vi "FeedbackDecode_20200902.vi"() -> ()   [LabVIEW 2016] (continued)
        n284 = call "FeedbackDecode_PlotHeatmap.vi"("Range"=w3234, "GridIntensity"=w3245, "Instance"=1, "Mode"=w3251) -> ("Pic"=w3236:picture)  [unwired: 2 in, 1 out]
        n285 = call "FeedbackDecode_PlotHeatmap.vi"("Range"=w3234, "GridIntensity"=w3238, "Instance"=2, "Mode"=w3251) -> ("Pic"=w3235:picture)  [unwired: 2 in, 1 out]
        n286 = local write "MedianHM"(w3237) -> ()
        n287 = local write "UlnarHM"(w3236) -> ()
        n288 = local write "EMGHM"(w3235) -> ()
        n289 = for {
          tunnel: w3178 -> [w3331] mode=indexing
          tunnel: [w3330] -> w3180 mode=indexing
          tunnel: w3179 -> [w3327]
          tunnel: w3177 -> [w3329] mode=indexing
          tunnel: [w3326] -> w3176 mode=indexing
          n290 = Build Array(w3331) -> (w3332:dbl[])
          n291 = Build Array(w3329) -> (w3328:dbl[])
          n292 = Bundle By Name("Y"=w3332, "t0"=w3327) -> (w3330:waveform(dbl))  [unwired: 1 in]
          n293 = Bundle By Name("Y"=w3328, "t0"=w3327) -> (w3326:waveform(dbl))  [unwired: 1 in]
        }
        "TASKA Pressure" <- w3180
        "TASKA IR" <- w3176
        n294 = global read "FeedbackDecode_Globals.vi" "FD_PupilClust"() -> (→"PupilClust":T11)
        n295 = case shown="True" w3183 {
          frame False {
          }
          frame True {
            n296 = call <vilib>:"Play Sound File.vi"("path"=path "C:/Windows/Media/Windows Critical Stop.wav") -> ()  [unwired: 9 in, 2 out]
          }
        }
        n297 = local read "CurrMvnt"() -> (w3317:T1)
        n298 = local read "MSMSSphere"() -> (w3270:dbl[][])
        n299 = local read "BaseCnt3"() -> (w3186:i64)
        n300 = local read "LoopCnt"() -> (w3210:u64)
        n301 = case shown="\"Training\"" w3207 {
          tunnel: w3231 -> [_ _ w3412]
          tunnel: [T26 {"[0]"=0.0, "[1]"=0.0, "[2]"=0.0, "[3]"=0.0, "[4]"=0.0, "[5]"=0.0, "[6]"=0.0, "[7]"=0.0, "[8]"=0.0, "[9]"=0.0, "[10]"=0.0, "[11]"=0.0} ("Kinematics") w3411 w3412] -> w3266
          tunnel: w3232 -> [_ w3411 _]
          frame "Off" {
          }
          frame "Training" {
          }
          frame "Decode", Default {
          }
        }
        n302 = local read "MSMSMvnt"() -> (w3271:dbl[])
        n303 = Unbundle By Name(w3317) -> ("Radius"=w3172:dbl)
        n304 = Equal?(x=w3210, y=w3186) -> (x = y?=w3211:bool)
        n305 = Replace Array Subset(array=w3270, new element=w3312, index (row)=0 ("disabled index (row)"), index (col)=0 ("disabled index (col)")) -> (w3174:dbl[][])
        n306 = Cluster To Array(cluster=w3266) -> (array=w3230:dbl[])
        n307 = case shown="True" w3211 {
          frame False {
          }
          frame True {
            n308 = local read "PulseStim"() -> (w3355:bool)
            n309 = case shown="True" w3355 {
              frame False {
                n310 = local read "EncodeClust"() -> (w3358:T9)
                n311 = local write "PulseStim"(TRUE ("PulseStim")) -> ()
                n312 = local read "EncodeClust"() -> (w3362:T9)
                n313 = Unbundle By Name(w3358) -> ("Wait Period"=w3359:dbl)
                n314 = Unbundle By Name(w3362) -> ("Pulse"=w3361:bool)
                n315 = local read "LoopCnt"() -> (w3357:u64)
                n316 = expression code="x*100"(w3359) -> (w3360:dbl)
                n317 = case shown="True" w3361 {
                  tunnel: ["SS.PulseStim=1;" ("EventStr") "SS.PulseStim=0;" ("EventStr")] -> w3364
                  frame False {
                  }
                  frame True {
                  }
                }
                n318 = Add(x=w3357, y=w3360) -> (x+y=w3356:dbl)
                n319 = local write "BaseCnt3"(w3356) -> ()
                n320 = local read "DecodeClust"() -> (w3365:T5)
                n321 = Bundle By Name(cluster=w3365, "EventStr"=w3364) -> (w3367:T5)
                n322 = call "FeedbackDecode_MLComCtrl.vi"("DecodeClustIn"=w3367, "Mode"=T19."SendEvent") -> ()  [unwired: 6 in, 4 out]
              }
              frame True {
                n323 = local read "EncodeClust"() -> (w3372:T9)
                n324 = local write "PulseStim"(FALSE ("PulseStim")) -> ()
                n325 = Unbundle By Name(w3372) -> ("Train Period"=w3373:dbl)
                n326 = local read "LoopCnt"() -> (w3371:u64)
                n327 = expression code="x*100"(w3373) -> (w3374:dbl)
                n328 = Add(x=w3371, y=w3374) -> (x+y=w3370:dbl)
                n329 = local read "DecodeClust"() -> (w3377:T5)
                n330 = local write "BaseCnt3"(w3370) -> ()
                n331 = Bundle By Name(cluster=w3377, "EventStr"="SS.PulseStim=1;") -> (w3379:T5)
                n332 = call "FeedbackDecode_MLComCtrl.vi"("DecodeClustIn"=w3379, "Mode"=T19."SendEvent") -> ()  [unwired: 6 in, 4 out]
              }
            }
          }
        }
        n333 = In Range and Coerce(upper limit=1.0, x=w3230, lower limit=-1.0) -> (coerced(x)=w3273:dbl[])  [unwired: 1 out]
        n334 = Unbundle By Name(w3215) -> ("CtrlButtons.HideSphrs"=w3218:bool)
        n335 = Initialize Array(w3172, 6 ("dimension size")) -> (w3170:dbl[])
        n336 = call "FeedbackDecode_InWindowMDim.vi"("Radius"=w3172, "Targ"=w3222, "Pos"=w3273) -> ("Status"=w3265:enum16{"In", "Out"}, "TargStatus"=w3269:i16[], "TargDist"=w3264:dbl[])  [unwired: 1 in, 1 out]
        n337 = case shown="\"Acquire Start\"" w3325 {
          tunnel: w3265 -> [_ w3511 w3584 _]
          frame "Initialize", Default {
            n338 = local read "DecodeClust"() -> (w3423:T5)
            n339 = Unbundle By Name(w3423) -> ("TestType"=w3421:T23, "CtrlButtons.StartTrials"=w3418:bool, "KinSrc"=w3422:T37)
            n340 = Equal?(x=T30."MSMS", y=w3421) -> (x = y?=w3419:bool)
            n341 = And(x=w3419, y=w3418) -> (x .and. y?=w3417:bool)
            n342 = case shown="True" w3417 {
              tunnel: w3422 -> [_ w3424]
              frame False {
              }
              frame True {
                n343 = stacked-sequence {
                  tunnel: w3424 -> [w3431 _]
                  frame #0 {
                    w3433 = enum16{"Initialize", "Reset", "Run"}."Initialize" ("Mode")
                    # "For step targets, the duration of step is set to ART+ARTR and ARD/ETD are a function of the hold and rise times of the movement."
                    n344 = local read "MvntBuilder"() -> (w3428:T6)
                    n345 = Unbundle By Name(w3428) -> ("MvntList"=w3446:T24)
                    n346 = Unbundle By Name(w3428) -> ("TargParams.Gain"=w3435:dbl, "TargParams.Acc"=w3451:dbl, "Mode"=w3447:enum16{"Selected", "Block", "Random"}, "NTrials"=w3449:dbl)
                    n347 = local read "Timing"() -> (w3455:T3)
                    n348 = Array Size(array=w3446) -> (size(s)=w3448:i32)
                    n349 = case shown="\"Block\", Default" w3447 {
                      selector: w3447 -> [_ w3461]
                      tunnel: [w3460 w3465] -> w3429
                      tunnel: w3448 -> [_ w3464]
                      tunnel: w3449 -> [_ w3463]
                      tunnel: [0.0 ("Perc") w3462] -> w3427
                      frame "Selected" {
                        n350 = property on="MvntList" class="Arr (strict)"() -> ("Index Values"=w3459:u32[])  [unwired: 2 in, 2 out]
                        n351 = Index Array(array=w3459) -> (element=w3460:u32)  [unwired: 1 in]
                      }
                      frame "Block", Default {
                        n352 = call "FeedbackDecode_GenRandBlockIdxs2.vi"("Mode"=w3461, "NumTrials"=w3463, "NumIdxs"=w3464) -> ("RandIdx"=w3465:dbl, "Perc"=w3462:dbl)  [unwired: 2 in]
                      }
                    }
                    "NextIdx" <- w3429
                    n353 = local read "LoopPeriod"() -> (w3434:u64)
                    n354 = Unbundle By Name(w3455) -> ("Dur.ART"=w3437:dbl, "Rnd.ARTR"=w3436:dbl)
                    n355 = Index Array(array=w3446, index=w3429) -> (element=w3425:T1)
                    n356 = Bundle By Name(cluster=w3428, "PercTrials"=w3427) -> (w3426:T6)
                    n357 = Unbundle By Name(w3425) -> ("Tracking"=w3440:enum8{"False", "True", "Mixed"})
                    n358 = Add(x=w3437, y=w3436) -> (x+y=w3438:dbl)
                    n359 = local write "CurrMvnt"(w3425) -> ()
                    n360 = Subtract(x=1.0, y=w3451) -> (x-y=w3453:dbl)
                    n361 = call "FeedbackDecode_GenContTarget.vi"("Gain"=w3435, "StepTime (ms)"=w3438, "MvntClust"=w3425, "LoopPeriod (ms)"=w3434, "Mode"=w3433) -> ()  [unwired: 1 in, 4 out]
                    n362 = call "FeedbackDecode_GenContMvnt.vi"("Mode"=w3433, "LoopPeriod"=w3434, "Gain"=w3435, "MvntClust"=w3425) -> ("MaxTimes (ms)"=w3439:T42)  [unwired: 2 in, 2 out]
                    n363 = local read "MvntEvnt"() -> (w3430:refnum<user-event>)
                    n364 = Unbundle By Name(w3439) -> ("Hold"=w3441:dbl, "Rise"=w3445:dbl, "Trial"=w3452:dbl)
                    n365 = Not Equal To 0?(x=w3440) -> (x != 0?=w3442:bool)
                    "Tracking" <- w3442
                    n366 = local write "MvntBuilder"(w3426) -> ()
                    n367 = Generate User Event(user event=w3430, event data cluster=w3429) -> ()  [unwired: 2 in, 2 out]
                    n368 = expression code="2*x"(w3445) -> (w3444:dbl)
                    n369 = Multiply(x=w3452, y=w3453) -> (x*y=w3454:dbl)
                    n370 = case shown="False" w3442 {
                      tunnel: w3455 -> [w3472 w3485]
                      tunnel: [w3471 w3484] -> w3432
                      tunnel: w3441 -> [w3470 _]
                      tunnel: w3444 -> [w3469 _]
                      tunnel: [w3466 w3482] -> w3443
                      tunnel: w3452 -> [w3467 w3482]
                      tunnel: w3431 -> [w3468 _]
                      tunnel: w3454 -> [_ w3481]
                      frame False {
                        n371 = case shown="\"Training\"" w3468 {
                          tunnel: w3472 -> [w3474 w3480]
                          tunnel: [w3474 w3479] -> w3471
                          tunnel: w3470 -> [_ w3478]
                          tunnel: w3469 -> [_ w3477]
                          tunnel: w3467 -> [w3473 w3476]
                          tunnel: [w3473 w3476] -> w3466
                          frame "Off", Default {
                          }
                          frame "Training" {
                            w3475 = u16 0 ("Rnd.ARDR")
                            n372 = Bundle By Name(cluster=w3480, "Rnd.ARDR"=w3475, "Dur.ARD"=w3478, "Dur.ETD"=w3477, "Rnd.ETDR"=w3475) -> (w3479:T3)
                          }
                        }
                      }
                      frame True {
                        n373 = Bundle By Name(cluster=w3485, "Rnd.ARTR"=u16 0, "Dur.ART"=w3482, "Dur.ETD"=w3481) -> (w3484:T3)
                      }
                    }
                    "TrialTime (ms)" <- w3443
                    n374 = local read "PrevIdx"() -> (w3456:dbl)
                    n375 = Not Equal?(x=w3429, y=w3456) -> (x != y?=w3457:bool)
                    n376 = case shown="True" w3457 {
                      tunnel: w3431 -> [_ w3490]
                      tunnel: w3432 -> [w3486 w3489]
                      frame False {
                        n377 = local write "iTiming"(w3486) -> ()
                      }
                      frame True {
                        n378 = case shown="\"Training\"" w3490 {
                          tunnel: w3489 -> [w3491 w3492]
                          frame "Off", Default {
                            n379 = local write "iTiming"(w3491) -> ()
                          }
                          frame "Training" {
                            n380 = Unbundle By Name(w3492) -> ("Dur.ASD"=w3495:dbl)
                            n381 = Multiply(x=w3495, y=u16 2) -> (x*y=w3496:dbl)
                            n382 = Bundle By Name(cluster=w3492, "Dur.ASD"=w3496) -> (w3493:T3)
                            n383 = local write "iTiming"(w3493) -> ()
                          }
                        }
                        n384 = local read "LoopCnt"() -> (w3487:u64)
                        n385 = local write "ResetCorr"(TRUE ("ResetCorr")) -> ()
                        n386 = local write "BaseCnt1"(w3487) -> ()
                      }
                    }
                  }
                  frame #1 {
                    n387 = local write "Outcome"(enum16{"---", "Success", "Failure"}."---" ("Outcome")) -> ()
                    n388 = local read "NextIdx"() -> (w3497:dbl)
                    n389 = local read "LoopCnt"() -> (w3507:u64)
                    n390 = call "FeedbackDecode_RunOnce.vi"("Instance"=0, "Mode"=enum16{"Reset", "Run"}."Reset") -> ()  [unwired: 1 out]
                    n391 = local write "PrevIdx"(w3497) -> ()
                    n392 = call "FeedbackDecode_LoopComp.vi"("LoopCount"=w3507, "Instance"=0, "Mode"=enum16{"Reset", "Run"}."Reset") -> ()  [unwired: 3 in, 2 out]
                    n393 = call "FeedbackDecode_RunOnce.vi"("Instance"=1, "Mode"=enum16{"Reset", "Run"}."Reset") -> ()  [unwired: 1 out]
                    n394 = local write "State"(T16."Acquire Start" ("Current State")) -> ()
                    "TargCnt" <- u64 0 ("TargAcc")
                    "SubCase" <- 0 ("SubCase")
                  }
                }
              }
            }
          }
          frame "Acquire Start" {
            n395 = local read "iTiming"() -> (w3514:T3)
            n396 = Unbundle By Name(w3514) -> ("Dur.ASD"=w3509:dbl, "Rnd.ASDR"=w3513:dbl)
            n397 = Equal To 0?(x=w3509) -> (x = 0?=w3510:bool)
            n398 = case shown="True" w3510 {
              tunnel: [w3515 enum16{"In", "Out"}."In" ("Status")] -> w3512
              tunnel: w3511 -> [w3515 _]
              frame False {
              }
              frame True {
              }
            }
            n399 = case shown="\"In\", Default" w3512 {
              tunnel: w3509 -> [w3518 _]
              tunnel: w3513 -> [w3517 _]
              frame "In", Default {
                n400 = local read "LoopPeriod"() -> (w3526:u64)
                n401 = local read "LoopCnt"() -> (w3523:u64)
                n402 = local read "Timing"() -> (w3519:T3)
                n403 = call "FeedbackDecode_LoopComp.vi"("RandTime"=w3517, "LoopPeriod"=w3526, "SetTime"=w3518, "LoopCount"=w3523, "Instance"=0, "Mode"=enum16{"Reset", "Run"}."Run") -> ("ActualTime"=w3521:u64, "Outcome"=w3520:enum16{"TimeIn", "TimeOut"})
                n404 = Bundle By Name(cluster=w3519, "Act.ASDA"=w3521) -> (w3522:T3)
                n405 = local write "Timing"(w3522) -> ()
                n406 = case shown="\"TimeOut\"" w3520 {
                  frame "TimeIn", Default {
                    n407 = local read "DecodeClust"() -> (w3528:T5)
                    n408 = Unbundle By Name(w3528) -> ("CtrlButtons.ResetTrial"=w3527:bool)
                    n409 = case shown="True" w3527 {
                      frame False {
                      }
                      frame True {
                        n410 = local read "LoopCnt"() -> (w3531:u64)
                        n411 = local write "State"(T16."Finalize" ("Current State")) -> ()
                        n412 = call "FeedbackDecode_RunOnce.vi"("Instance"=0, "Mode"=enum16{"Reset", "Run"}."Reset") -> ()  [unwired: 1 out]
                        n413 = call "FeedbackDecode_LoopComp.vi"("LoopCount"=w3531, "Instance"=0, "Mode"=enum16{"Reset", "Run"}."Reset") -> ()  [unwired: 3 in, 2 out]
                      }
                    }
                  }
                  frame "TimeOut" {
                    n414 = local read "SubCase"() -> (w3535:i32)
                    n415 = case shown="1, Default" w3535 {
                      frame 0 {
                        # "This subcase delays the execution by 1 loop iteration"
                        n416 = local read "DecodeClust"() -> (w3538:T5)
                        n417 = Unbundle By Name(w3538) -> ("CtrlButtons.CalDEKA"=w3537:bool)
                        n418 = local write "SubCase"(1 ("SubCase")) -> ()
                        n419 = case shown="True" w3537 {
                          frame False {
                          }
                          frame True {
                            n420 = property on="HideSphrs" class="Bool (strict)"("Val(Sgnl)"=TRUE ("Value (Signaling)")) -> ()  [unwired: 2 in, 2 out]
                          }
                        }
                      }
                      frame 1, Default {
                        n421 = local read "LoopCnt"() -> (w3554:u64)
                        n422 = local read "LoopCnt"() -> (w3557:u64)
                        n423 = local read "NIPTime"() -> (w3544:dbl)
                        n424 = local read "LoopCnt"() -> (w3549:u64)
                        n425 = call "FeedbackDecode_GenContTarget.vi"("LoopCount"=w3554, "Mode"=enum16{"Initialize", "Reset", "Run"}."Reset") -> ()  [unwired: 4 in, 4 out]
                        n426 = call "FeedbackDecode_GenContMvnt.vi"("Mode"=enum16{"Initialize", "Reset", "Run"}."Reset", "LoopCount"=w3557) -> ()  [unwired: 4 in, 3 out]
                        n427 = local read "LoopCnt"() -> (w3563:u64)
                        n428 = Format Into String(w3549) -> (resulting string=w3541:string)  [unwired: 3 in, 1 out]
                        n429 = call-poly "FeedbackDecode_VariablesToString.vi"("Format"="%0.0f", "ValueIn"=w3544, "FieldName"="NIPTime" ("Key Word")) -> ("StringOut"=w3547:string)  [unwired: 4 in]
                        n430 = local read "EventParamsFID"() -> (w3543:refnum<file>)
                        n431 = Concatenate Strings("TargOn:SS.EventID=" ("string"), w3541) -> (w3546:string)
                        n432 = call "FeedbackDecode_LoopComp.vi"("LoopCount"=w3563, "Instance"=0, "Mode"=enum16{"Reset", "Run"}."Reset") -> ()  [unwired: 3 in, 2 out]
                        n433 = Concatenate Strings(w3546, ";" ("string"), w3547) -> (w3540:string)
                        n434 = call "FeedbackDecode_WriteTextEOL.vi"("text"=w3540, "refnum in"=w3543) -> ()  [unwired: 8 in, 2 out]
                        n435 = local read "DecodeClust"() -> (w3553:T5)
                        n436 = Bundle By Name(cluster=w3553, "EventStr"=w3540) -> (w3551:T5)
                        n437 = local read "LoopCnt"() -> (w3560:u64)
                        n438 = call "FeedbackDecode_MLComCtrl.vi"("DecodeClustIn"=w3551, "Mode"=T19."SendEvent") -> ()  [unwired: 6 in, 4 out]
                        n439 = local write "State"(T16."Acquire Response" ("Current State")) -> ()
                        n440 = call "FeedbackDecode_LoopComp.vi"("LoopCount"=w3560, "Instance"=1, "Mode"=enum16{"Reset", "Run"}."Reset") -> ()  [unwired: 3 in, 2 out]
                      }
                    }
                  }
                }
              }
              frame "Out" {
                n441 = local read "LoopCnt"() -> (w3569:u64)
                n442 = call "FeedbackDecode_LoopComp.vi"("LoopCount"=w3569, "Instance"=0, "Mode"=enum16{"Reset", "Run"}."Reset") -> ()  [unwired: 3 in, 2 out]
                n443 = local read "DecodeClust"() -> (w3566:T5)
                n444 = Unbundle By Name(w3566) -> ("CtrlButtons.ResetTrial"=w3565:bool)
                n445 = case shown="True" w3565 {
                  frame False {
                  }
                  frame True {
                    n446 = call "FeedbackDecode_RunOnce.vi"("Instance"=0, "Mode"=enum16{"Reset", "Run"}."Reset") -> ()  [unwired: 1 out]
                    n447 = local write "State"(T16."Finalize" ("Current State")) -> ()
                  }
                }
              }
            }
          }
          frame "Acquire Response" {
            n448 = local read "Timing"() -> (w3573:T3)
            n449 = local read "iTiming"() -> (w3579:T3)
            n450 = local read "LoopPeriod"() -> (w3575:u64)
            n451 = local read "LoopCnt"() -> (w3578:u64)
            n452 = Unbundle By Name(w3579) -> ("Dur.ART"=w3581:dbl, "Rnd.ARTR"=w3582:dbl)
            n453 = call "FeedbackDecode_LoopComp.vi"("RandTime"=w3582, "LoopPeriod"=w3575, "SetTime"=w3581, "LoopCount"=w3578, "Instance"=1, "Mode"=enum16{"Reset", "Run"}."Run") -> ("ActualTime"=w3583:u64, "Outcome"=w3574:enum16{"TimeIn", "TimeOut"})
            n454 = Bundle By Name(cluster=w3573, "Act.ARTA"=w3583) -> (w3580:T3)
            n455 = local write "Timing"(w3580) -> ()
            n456 = case shown="\"TimeOut\"" w3574 {
              tunnel: w3584 -> [w3585 _]
              frame "TimeIn", Default {
                n457 = case shown="\"Out\"" w3585 {
                  frame "In", Default {
                    n458 = local read "Tracking"() -> (w3586:bool)
                    n459 = case shown="False" w3586 {
                      tunnel: [w3589 w3601] -> w3587
                      frame False {
                        n460 = local read "Timing"() -> (w3588:T3)
                        n461 = local read "iTiming"() -> (w3594:T3)
                        n462 = local read "LoopPeriod"() -> (w3598:u64)
                        n463 = local read "LoopCnt"() -> (w3595:u64)
                        n464 = Unbundle By Name(w3594) -> ("Dur.ARD"=w3592:dbl, "Rnd.ARDR"=w3591:dbl)
                        n465 = call "FeedbackDecode_LoopComp.vi"("RandTime"=w3591, "LoopPeriod"=w3598, "SetTime"=w3592, "LoopCount"=w3595, "Instance"=0, "Mode"=enum16{"Reset", "Run"}."Run") -> ("ActualTime"=w3590:u64, "Outcome"=w3589:enum16{"TimeIn", "TimeOut"})
                        n466 = Bundle By Name(cluster=w3588, "Act.ARDA"=w3590) -> (w3593:T3)
                        n467 = local write "Timing"(w3593) -> ()
                      }
                      frame True {
                        n468 = local read "TargCnt"() -> (w3602:u64)
                        n469 = local read "MvntBuilder"() -> (w3600:T6)
                        n470 = local read "TrialTime (ms)"() -> (w3606:dbl)
                        n471 = local read "LoopPeriod"() -> (w3604:u64)
                        n472 = Increment(x=w3602) -> (x+1=w3603:u64)
                        n473 = Unbundle By Name(w3600) -> ("TargParams.Acc"=w3599:dbl)
                        n474 = Multiply(x=w3603, y=w3604) -> (x*y=w3607:u64)
                        n475 = Multiply(x=w3606, y=w3599) -> (x*y=w3605:dbl)
                        n476 = local write "TargCnt"(w3603) -> ()
                        n477 = Greater Or Equal?(x=w3607, y=w3605) -> (x >= y?=w3608:bool)
                        n478 = Boolean To (0,1)(Boolean=w3608) -> (0, 1=w3601:i16)
                      }
                    }
                    n479 = case shown="0, Default" w3587 {
                      frame 0, Default {
                        # "TimeIn"
                        n480 = local read "DecodeClust"() -> (w3610:T5)
                        n481 = Unbundle By Name(w3610) -> ("CtrlButtons.ResetTrial"=w3609:bool)
                        n482 = call "FeedbackDecode_RunOnce.vi"("Instance"=0, "Mode"=enum16{"Reset", "Run"}."Run") -> ("State"=w3613:enum16{"RunOnce", "Finished"})
                        n483 = case shown="\"RunOnce\", Default" w3613 {
                          tunnel: w3609 -> [_ w3627]
                          frame "RunOnce", Default {
                            n484 = local read "NIPTime"() -> (w3619:dbl)
                            n485 = local read "LoopCnt"() -> (w3625:u64)
                            n486 = Format Into String(w3625) -> (resulting string=w3616:string)  [unwired: 3 in, 1 out]
                            n487 = call-poly "FeedbackDecode_VariablesToString.vi"("Format"="%0.0f", "ValueIn"=w3619, "FieldName"="NIPTime" ("Key Word")) -> ("StringOut"=w3622:string)  [unwired: 4 in]
                            n488 = local read "EventParamsFID"() -> (w3618:refnum<file>)
                            n489 = Concatenate Strings("InTarg:SS.EventID=" ("string"), w3616) -> (w3621:string)
                            n490 = Concatenate Strings(w3621, ";" ("string"), w3622) -> (w3623:string)
                            n491 = call "FeedbackDecode_WriteTextEOL.vi"("text"=w3623, "refnum in"=w3618) -> ()  [unwired: 8 in, 2 out]
                          }
                          frame "Finished" {
                            n492 = case shown="False" w3627 {
                              frame False {
                              }
                              frame True {
                                n493 = local read "LoopCnt"() -> (w3628:u64)
                                n494 = call "FeedbackDecode_LoopComp.vi"("LoopCount"=w3628, "Instance"=0, "Mode"=enum16{"Reset", "Run"}."Reset") -> ()  [unwired: 3 in, 2 out]
                                n495 = local write "State"(T16."Finalize" ("Current State")) -> ()
                                n496 = call "FeedbackDecode_RunOnce.vi"("Instance"=0, "Mode"=enum16{"Reset", "Run"}."Reset") -> ()  [unwired: 1 out]
                              }
                            }
                          }
                        }
                        n497 = call "FeedbackDecode_RunOnce.vi"("Instance"=1, "Mode"=enum16{"Reset", "Run"}."Reset") -> ()  [unwired: 1 out]
                      }
                      frame 1 {
                        # "TimeOut"
                        n498 = local read "LoopCnt"() -> (w3649:u64)
                        n499 = call "FeedbackDecode_LoopComp.vi"("LoopCount"=w3649, "Instance"=1, "Mode"=enum16{"Reset", "Run"}."Reset") -> ()  [unwired: 3 in, 2 out]
                        n500 = call "FeedbackDecode_RunOnce.vi"("Instance"=0, "Mode"=enum16{"Reset", "Run"}."Reset") -> ()  [unwired: 1 out]
                        n501 = local read "LoopCnt"() -> (w3656:u64)
                        n502 = call "FeedbackDecode_LoopComp.vi"("LoopCount"=w3656, "Instance"=0, "Mode"=enum16{"Reset", "Run"}."Reset") -> ()  [unwired: 3 in, 2 out]
                        n503 = local write "State"(T16."Finalize" ("Current State")) -> ()
                        n504 = local read "NIPTime"() -> (w3641:dbl)
                        n505 = local read "LoopCnt"() -> (w3646:u64)
                        n506 = local write "Outcome"(enum16{"---", "Success", "Failure"}."Success" ("Outcome")) -> ()
                        n507 = Format Into String(w3646) -> (resulting string=w3638:string)  [unwired: 3 in, 1 out]
                        n508 = call-poly "FeedbackDecode_VariablesToString.vi"("Format"="%0.0f", "ValueIn"=w3641, "FieldName"="NIPTime" ("Key Word")) -> ("StringOut"=w3644:string)  [unwired: 4 in]
                        n509 = local read "EventParamsFID"() -> (w3640:refnum<file>)
                        n510 = Concatenate Strings("Success:SS.EventID=" ("string"), w3638) -> (w3643:string)
                        n511 = Concatenate Strings(w3643, ";" ("string"), w3644) -> (w3634:string)
                        n512 = call "FeedbackDecode_WriteTextEOL.vi"("text"=w3634, "refnum in"=w3640) -> ()  [unwired: 8 in, 2 out]
                        n513 = local read "DecodeClust"() -> (w3637:T5)
                        n514 = Bundle By Name(cluster=w3637, "EventStr"=w3634) -> (w3635:T5)
                        n515 = call "FeedbackDecode_MLComCtrl.vi"("DecodeClustIn"=w3635, "Mode"=T19."SendEvent") -> ()  [unwired: 6 in, 4 out]
                      }
                    }
                  }
                  frame "Out" {
                    n516 = local read "DecodeClust"() -> (w3659:T5)
                    n517 = Unbundle By Name(w3659) -> ("CtrlButtons.ResetTrial"=w3658:bool)
                    n518 = case shown="True" w3658 {
                      frame False {
                      }
                      frame True {
                        n519 = local write "State"(T16."Finalize" ("Current State")) -> ()
                      }
                    }
                    n520 = local read "LoopCnt"() -> (w3667:u64)
                    n521 = call "FeedbackDecode_LoopComp.vi"("LoopCount"=w3667, "Instance"=0, "Mode"=enum16{"Reset", "Run"}."Reset") -> ()  [unwired: 3 in, 2 out]
                    n522 = call "FeedbackDecode_RunOnce.vi"("Instance"=1, "Mode"=enum16{"Reset", "Run"}."Run") -> ("State"=w3662:enum16{"RunOnce", "Finished"})
                    n523 = call "FeedbackDecode_RunOnce.vi"("Instance"=0, "Mode"=enum16{"Reset", "Run"}."Reset") -> ()  [unwired: 1 out]
                    n524 = case shown="\"RunOnce\", Default" w3662 {
                      frame "RunOnce", Default {
                        n525 = local read "NIPTime"() -> (w3671:dbl)
                        n526 = local read "LoopCnt"() -> (w3677:u64)
                        n527 = Format Into String(w3677) -> (resulting string=w3668:string)  [unwired: 3 in, 1 out]
                        n528 = call-poly "FeedbackDecode_VariablesToString.vi"("Format"="%0.0f", "ValueIn"=w3671, "FieldName"="NIPTime" ("Key Word")) -> ("StringOut"=w3674:string)  [unwired: 4 in]
                        n529 = local read "EventParamsFID"() -> (w3670:refnum<file>)
                        n530 = Concatenate Strings("OutTarg:SS.EventID=" ("string"), w3668) -> (w3673:string)
                        n531 = Concatenate Strings(w3673, ";" ("string"), w3674) -> (w3675:string)
                        n532 = call "FeedbackDecode_WriteTextEOL.vi"("text"=w3675, "refnum in"=w3670) -> ()  [unwired: 8 in, 2 out]
                      }
                      frame "Finished" {
                      }
                    }
                  }
                }
              }
              frame "TimeOut" {
                n533 = local read "LoopCnt"() -> (w3702:u64)
                n534 = local read "LoopCnt"() -> (w3695:u64)
                n535 = call "FeedbackDecode_RunOnce.vi"("Instance"=0, "Mode"=enum16{"Reset", "Run"}."Reset") -> ()  [unwired: 1 out]
                n536 = call "FeedbackDecode_LoopComp.vi"("LoopCount"=w3702, "Instance"=0, "Mode"=enum16{"Reset", "Run"}."Reset") -> ()  [unwired: 3 in, 2 out]
                n537 = call "FeedbackDecode_LoopComp.vi"("LoopCount"=w3695, "Instance"=1, "Mode"=enum16{"Reset", "Run"}."Reset") -> ()  [unwired: 3 in, 2 out]
                n538 = local write "Outcome"(enum16{"---", "Success", "Failure"}."Failure" ("Outcome")) -> ()
                n539 = local write "State"(T16."Finalize" ("Current State")) -> ()
                n540 = local read "NIPTime"() -> (w3687:dbl)
                n541 = local read "LoopCnt"() -> (w3692:u64)
                n542 = Format Into String(w3692) -> (resulting string=w3684:string)  [unwired: 3 in, 1 out]
                n543 = call-poly "FeedbackDecode_VariablesToString.vi"("Format"="%0.0f", "ValueIn"=w3687, "FieldName"="NIPTime" ("Key Word")) -> ("StringOut"=w3690:string)  [unwired: 4 in]
                n544 = local read "EventParamsFID"() -> (w3686:refnum<file>)
                n545 = Concatenate Strings("Failure:SS.EventID=" ("string"), w3684) -> (w3689:string)
                n546 = Concatenate Strings(w3689, ";" ("string"), w3690) -> (w3680:string)
                n547 = call "FeedbackDecode_WriteTextEOL.vi"("text"=w3680, "refnum in"=w3686) -> ()  [unwired: 8 in, 2 out]
                n548 = local read "DecodeClust"() -> (w3683:T5)
                n549 = Bundle By Name(cluster=w3683, "EventStr"=w3680) -> (w3681:T5)
                n550 = call "FeedbackDecode_MLComCtrl.vi"("DecodeClustIn"=w3681, "Mode"=T19."SendEvent") -> ()  [unwired: 6 in, 4 out]
              }
            }
          }
          frame "Finalize" {
            # "End of trial delay"
            n551 = local read "Timing"() -> (w3704:T3)
            n552 = local read "iTiming"() -> (w3708:T3)
            n553 = local read "LoopPeriod"() -> (w3711:u64)
            n554 = local read "LoopCnt"() -> (w3714:u64)
            n555 = Unbundle By Name(w3708) -> ("Dur.ETD"=w3707:dbl, "Rnd.ETDR"=w3706:dbl)
            n556 = call "FeedbackDecode_LoopComp.vi"("RandTime"=w3706, "LoopPeriod"=w3711, "SetTime"=w3707, "LoopCount"=w3714, "Instance"=0, "Mode"=enum16{"Reset", "Run"}."Run") -> ("ActualTime"=w3705:u64, "Outcome"=w3710:enum16{"TimeIn", "TimeOut"})
            n557 = Bundle By Name(cluster=w3704, "Act.ETDA"=w3705) -> (w3709:T3)
            n558 = local write "Timing"(w3709) -> ()
            n559 = case shown="\"TimeOut\"" w3710 {
              frame "TimeIn", Default {
                n560 = call "FeedbackDecode_RunOnce.vi"("Instance"=0, "Mode"=enum16{"Reset", "Run"}."Run") -> ("State"=w3715:enum16{"RunOnce", "Finished"})
                n561 = case shown="\"RunOnce\", Default" w3715 {
                  frame "RunOnce", Default {
                    n562 = local read "DecodeClust"() -> (w3721:T5)
                    n563 = Unbundle By Name(w3721) -> ("CtrlButtons.CalDEKA"=w3720:bool)
                    n564 = case shown="True" w3720 {
                      frame False {
                      }
                      frame True {
                        n565 = property on="HideSphrs" class="Bool (strict)"("Val(Sgnl)"=FALSE ("Value (Signaling)")) -> ()  [unwired: 2 in, 2 out]
                      }
                    }
                    n566 = call "FeedbackDecode_GenContTarget.vi"("LoopCount"=-inf, "Mode"=enum16{"Initialize", "Reset", "Run"}."Reset") -> ()  [unwired: 4 in, 4 out]
                    n567 = local read "Outcome"() -> (w3722:enum16{"---", "Success", "Failure"})
                    n568 = case shown="\"Failure\"" w3722 {
                      frame "---", Default {
                      }
                      frame "Success" {
                        n569 = local read "PSRef"() -> (w3727:refnum<vi>)
                        n570 = call-by-ref "Start Asynchronous Call"(reference=w3727, "Mode"=enum16{"Cue", "Success", "Failure", "Abort"}."Success", "#S"=1000.0, "Fs"=5000.0) -> ()  [unwired: 10 in, 2 out]
                      }
                      frame "Failure" {
                        n571 = local read "PSRef"() -> (w3731:refnum<vi>)
                        n572 = call-by-ref "Start Asynchronous Call"(reference=w3731, "Mode"=enum16{"Cue", "Success", "Failure", "Abort"}."Failure", "#S"=1000.0 ("Volume"), "Fs"=5000.0) -> ()  [unwired: 10 in, 2 out]
                      }
                    }
                  }
                  frame "Finished" {
                  }
                }
              }
              frame "TimeOut" {
                n573 = local read "DecodeClust"() -> (w3741:T5)
                n574 = local read "MvntBuilder"() -> (w3732:T6)
                n575 = local read "CurrMvnt"() -> (w3739:T1)
                n576 = local read "Outcome"() -> (w3743:enum16{"---", "Success", "Failure"})
                n577 = call "FeedbackDecode_UpdateTrialCnt.vi"("DecodeClustIn"=w3741, "CurrMvnt"=w3739) -> ("DecodeClustOut"=w3740:T5)  [unwired: 1 in]
                n578 = Bundle By Name(cluster=w3740, "Outcome"=w3743) -> (w3742:T5)
                n579 = local read "Timing"() -> (w3756:T3)
                n580 = Unbundle By Name(w3732) -> ("TargParams"=w3757:cluster{"Gain":dbl, "Radius":dbl, "Acc":dbl})
                n581 = local read "EncodeClust"() -> (w3746:T9)
                n582 = local read "TrialArray"() -> (w3755:string[])
                n583 = local read "LoopCnt"() -> (w3737:u64)
                n584 = local read "NIPTime"() -> (w3738:dbl)
                n585 = call "FeedbackDecode_FPPNS2NIP.vi"("NIPTime"=w3738, "EncodeClust"=w3746, "LoopCnt"=w3737, "DecodeClust"=w3742, "TrialTiming"=w3756, "TargParams"=w3757, "MvntClust"=w3739) -> ("TrialParams"=w3748:string)  [unwired: 4 in]
                n586 = Match Pattern(string=w3748, regular expression="SS.MvntMat=\\[[-0-9,;\\.]+\\];") -> (match substring=w3753:string)  [unwired: 1 in, 3 out]
                n587 = local read "EventParamsFID"() -> (w3747:refnum<file>)
                n588 = Insert Into Array(array=w3755, new element=w3748) -> (w3754:string[])  [unwired: 1 in]
                n589 = Concatenate Strings("EndTrial:" ("String"), w3753) -> (w3749:string)
                n590 = Bundle By Name(cluster=w3742, "EventStr"=w3749) -> (w3745:T5)
                n591 = local write "TrialArray"(w3754) -> ()
                n592 = Unbundle By Name(w3732) -> ("PercTrials"=w3733:dbl)
                n593 = call "FeedbackDecode_WriteTextEOL.vi"("text"=w3748, "refnum in"=w3747) -> ()  [unwired: 8 in, 2 out]
                n594 = call "FeedbackDecode_MLComCtrl.vi"("DecodeClustIn"=w3745, "Mode"=T19."SendEvent") -> ("DecodeClustOut"=w3744:T5)  [unwired: 6 in, 3 out]
                n595 = Equal?(x=w3733, y=1.0) -> (x = y?=w3734:bool)
                n596 = Unbundle By Name(w3744) -> ("CtrlButtons.ResetTrial"=w3736:bool)
                n597 = case shown="False" w3736 {
                  tunnel: w3744 -> [w3760 w3795]
                  tunnel: w3734 -> [w3761 _]
                  tunnel: w3732 -> [w3759 _]
                  frame False {
                    n598 = case shown="True" w3761 {
                      tunnel: w3759 -> [_ w3766]
                      tunnel: w3760 -> [w3762 w3765]
                      frame False {
                        n599 = local write "DecodeClust"(w3762) -> ()
                      }
                      frame True {
                        n600 = flat-sequence {
                          tunnel: w3766 -> [w3769]
                          tunnel: w3765 -> [w3772]
                          tunnel: [w3771] -> w3764
                          tunnel: [w3770] -> w3763
                          tunnel: w3764 -> [w3782]
                          tunnel: w3763 -> [w3781]
                          frame #0 {
                            n601 = Unbundle By Name(w3769) -> ("Mode"=w3778:enum16{"Selected", "Block", "Random"}, "NTrials"=w3776:dbl, "MvntList"=w3775:T24)
                            n602 = local write "DecodeClust"(w3772) -> ()
                            n603 = Unbundle By Name(w3772) -> ("CtrlButtons.AcqTraining"=w3771:bool, "CtrlButtons.StartTrials"=w3770:bool)
                            n604 = Array Size(array=w3775) -> (size(s)=w3774:i32)
                            n605 = call "FeedbackDecode_GenRandBlockIdxs2.vi"("Mode"=w3778, "Reset"=TRUE, "NumTrials"=w3776, "NumIdxs"=w3774, "CurrIdx"=0.0) -> ("Perc"=w3768:dbl)  [unwired: 1 out]
                            n606 = Bundle By Name(cluster=w3769, "PercTrials"=w3768) -> (w3767:T6)
                            n607 = local write "MvntBuilder"(w3767) -> ()
                          }
                          frame #1 {
                            n608 = Build Array(w3782, w3781) -> (w3780:bool[])
                            n609 = Boolean Array To Number(Boolean array=w3780) -> (number=w3779:u32)
                            n610 = case shown="3" w3779 {
                              frame 0, Default {
                              }
                              frame 1 {
                                n611 = local read "MvntEvnt"() -> (w3783:refnum<user-event>)
                                n612 = property on="AcqTraining" class="Bool (strict)"("Val(Sgnl)"=FALSE ("Value (Signaling)")) -> ()  [unwired: 2 in, 2 out]
                                n613 = Generate User Event(user event=w3783, event data cluster=0.0 ("event data")) -> ()  [unwired: 2 in, 2 out]
                              }
                              frame 2 {
                                n614 = local read "MvntEvnt"() -> (w3786:refnum<user-event>)
                                n615 = property on="StartTrials" class="Bool (strict)"("Val(Sgnl)"=FALSE ("Value (Signaling)")) -> ()  [unwired: 2 in, 2 out]
                                n616 = Generate User Event(user event=w3786, event data cluster=0.0 ("event data")) -> ()  [unwired: 2 in, 2 out]
                              }
                              frame 3 {
                                w3792 = FALSE ("Value (Signaling)")
                                n617 = local read "MvntEvnt"() -> (w3789:refnum<user-event>)
                                n618 = property on="StartTrials" class="Bool (strict)"("Value"=w3792) -> (error out=w3791:errorcluster)  [unwired: 2 in, 1 out]
                                n619 = property on="AcqTraining" class="Bool (strict)"(error in=w3791, "Val(Sgnl)"=w3792) -> ()  [unwired: 1 in, 2 out]
                                n620 = Generate User Event(user event=w3789, event data cluster=0.0 ("event data")) -> ()  [unwired: 2 in, 2 out]
                              }
                            }
                          }
                        }
                      }
                    }
                  }
                  frame True {
                    n621 = Bundle By Name(cluster=w3795, "CtrlButtons.ResetTrial"=FALSE) -> (w3793:T5)
                    n622 = local write "DecodeClust"(w3793) -> ()
                  }
                }
                n623 = local write "State"(T16."Initialize" ("Current State")) -> ()
              }
            }
          }
        }
        n624 = Replace Array Subset(array=w3271, new element=w3273) -> (w3206:dbl[])  [unwired: 1 in]
        n625 = Replace Array Subset(array=w3174, new element=w3170, index (col)=3 ("disabled index (col)")) -> (w3173:dbl[][])  [unwired: 1 in]
        n626 = Replace Array Subset(array=w3173, new element=w3269, index (col)=4 ("disabled index (col)")) -> (w3220:dbl[][])  [unwired: 1 in]
        n627 = local write "Status"(w3265) -> ()
        n628 = local write "MSMSMvnt"(w3206) -> ()
        n629 = local write "TargDist"(w3264) -> ()
        n630 = case shown="True" w3218 {
          tunnel: w3220 -> [w3381 w3385]
          tunnel: [w3380 w3384] -> w3219
          frame False {
            n631 = Replace Array Subset(array=w3381, new element=dbl[] [1.0, 1.0, 1.0, 1.0, 1.0, 1.0] ("new element/subarray"), index (col)=5 ("disabled index (col)")) -> (w3380:dbl[][])  [unwired: 1 in]
          }
          frame True {
            n632 = Replace Array Subset(array=w3385, new element=dbl[] [0.0, 0.0, 0.0, 0.0, 0.0, 0.0] ("new element/subarray"), index (col)=5 ("disabled index (col)")) -> (w3384:dbl[][])  [unwired: 1 in]
          }
        }
        n633 = Unbundle By Name(w3209) -> ("CtrlButtons.ConnDEKA"=w3208:bool, "KMvntClust.CtrlMode"=w3205:T43, "KMvntClust.CtrlSpd"=w3201:sgl[], "KinSrc"=w3199:T37, "DEKAMode"=w3195:enum16{"Velocity", "Position"}, "CtrlButtons.CalDEKA"=w3202:bool)
        n634 = global write "FeedbackDecode_Globals.vi" "FD_MSMSMvnt"(w3206) -> ()
        n635 = call "FeedbackDecode_CombineMSMSPackets.vi"("SphereArray"=w3219, "MvntArray"=w3206) -> ()  [unwired: 1 in]
        n636 = local write "MSMSSphere"(w3219) -> ()
        n637 = case shown="False" w3202 {
          tunnel: w3202 -> [_ w3350]
          frame False {
          }
          frame True {
            n638 = call "FeedbackDecode_RunOnce.vi"("Instance"=2, "Mode"=enum16{"Reset", "Run"}."Run") -> ("State"=w3351:enum16{"RunOnce", "Finished"})
            n639 = case shown="\"RunOnce\", Default" w3351 {
              tunnel: w3350 -> [w3354 _]
              frame "RunOnce", Default {
                n640 = global write "FeedbackDecode_Globals.vi" "FD_CalDEKA"(w3354) -> ()
              }
              frame "Finished" {
              }
            }
          }
        }
        n641 = global write "FeedbackDecode_Globals.vi" "FD_ConnDEKA"(w3208) -> ()
        n642 = global write "FeedbackDecode_Globals.vi" "FD_CtrlMode"(w3205) -> ()
        n643 = global write "FeedbackDecode_Globals.vi" "FD_CtrlSpeed"(w3201) -> ()
        n644 = global write "FeedbackDecode_Globals.vi" "FD_KinSrc"(w3199) -> ()
        n645 = global write "FeedbackDecode_Globals.vi" "FD_DEKAMode"(w3195) -> ()
        n646 = global read "FeedbackDecode_Globals.vi" "FD_Stop"() -> (w3200:bool)
        n647 = node-c288() -> ()  [unwired: 1 in, 1 out]
        "LoopCnt" <- w3318
      }
      n648 = control-ref of="RespStr"() -> (w326:refnum<vi>)
      n649 = call "FeedbackDecode_PickROI.vi"("RespStrRef"=w326) -> ()  [unwired: 3 in]
      n650 = call "FeedbackDecode_PickROI_Adv.vi"("RespStrRef"=w326) -> ()  [unwired: 3 in]
      n651 = local read "PupilTracker"() -> (w325:bool)
      n652 = while {
        stop <- w336 stop-if-true
        n653 = Wait (ms)(milliseconds to wait=u32 1000) -> ()  [unwired: 1 out]
        n654 = local read "DataPath"() -> (w335:path)
        n655 = global read "FeedbackDecode_Globals.vi" "FD_Stop"() -> (w336:bool)
        n656 = call "FeedbackDecode_RecordAV.vi"("FullDataPath"=w335) -> ()  [unwired: 3 in]
      }
      n657 = case shown="True" w325 {
        frame False {
        }
        frame True {
          n658 = while {
            stop <- w330 stop-if-true
            n659 = local read "DataPath"() -> (w329:path)
            n660 = Wait (ms)(milliseconds to wait=u32 1000) -> ()  [unwired: 1 out]
            n661 = global read "FeedbackDecode_Globals.vi" "FD_Stop"() -> (w330:bool)
            n662 = call "FeedbackDecode_GetPupilInfo.vi"("FullDataPath"=w329) -> ()  [unwired: 3 in]
          }
        }
      }
      n663 = while {
        stop <- w339 stop-if-true
        n664 = local read "EvntReg"() -> (w338:refnum<event-registration>)
        n665 = event shown="[12] \"CognitiveLoad.ConnectECG\": Value Change" {
          selector: w338 -> [_ _ _ _ _ _ _ _ _ _ _ _ _ _ _ _ _ _ _ _ _ _ _ _ _ _ _ _ _ _ _ _ _ _ _ _ _ _ _ _ _ _ _ _ _ _ _ _ _ _ _ _ _ _ _ _ _ _ _ _ _ _ _ _ _ _ _ _ _ _ _ _ _ _ _ _ _ _ _ _ _ _ _ _ _ _ _ _ _ _ _ _ _ _ _ _ _ _ _ _ _ _ _ _ _ _ _ _ _ _ _ _]
          dyn-events: _ -> [_ _ _ _ _ _ _ _ _ _ _ _ _ _ _ _ _ _ _ _ _ _ _ _ _ _ _ _ _ _ _ _ _ _ _ _ _ _ _ _ _ _ _ _ _ _ _ _ _ _ _ _ _ _ _ _ _ _ _ _ _ _ _ _ _ _ _ _ _ _ _ _ _ _ _ _ _ _ _ _ _ _ _ _ _ _ _ _ _ _ _ _ _ _ _ _ _ _ _ _ _ _ _ _ _ _ _ _ _ _ _ _]
          timeout: _ -> [_ _ _ _ _ _ _ _ _ _ _ _ _ _ _ _ _ _ _ _ _ _ _ _ _ _ _ _ _ _ _ _ _ _ _ _ _ _ _ _ _ _ _ _ _ _ _ _ _ _ _ _ _ _ _ _ _ _ _ _ _ _ _ _ _ _ _ _ _ _ _ _ _ _ _ _ _ _ _ _ _ _ _ _ _ _ _ _ _ _ _ _ _ _ _ _ _ _ _ _ _ _ _ _ _ _ _ _ _ _ _ _]
          tunnel: [FALSE ("NewVal") FALSE ("NewVal") FALSE ("NewVal") w363 FALSE ("NewVal") FALSE ("NewVal") FALSE ("NewVal") FALSE ("NewVal") FALSE ("NewVal") FALSE ("NewVal") FALSE ("NewVal") FALSE ("NewVal") FALSE ("NewVal") FALSE ("NewVal") FALSE ("NewVal") FALSE ("NewVal") FALSE ("NewVal") FALSE ("NewVal") FALSE ("NewVal") FALSE ("NewVal") FALSE ("NewVal") FALSE ("NewVal") FALSE ("NewVal") FALSE ("NewVal") FALSE ("NewVal") FALSE ("NewVal") FALSE ("NewVal") FALSE ("NewVal") FALSE ("NewVal") FALSE ("NewVal") FALSE ("NewVal") FALSE ("NewVal") w1156 FALSE ("NewVal") FALSE ("NewVal") FALSE ("NewVal") FALSE ("NewVal") FALSE ("NewVal") FALSE ("NewVal") FALSE ("NewVal") FALSE ("NewVal") FALSE ("NewVal") FALSE ("NewVal") FALSE ("NewVal") FALSE ("NewVal") FALSE ("NewVal") FALSE ("NewVal") FALSE ("NewVal") FALSE ("NewVal") FALSE ("NewVal") FALSE ("NewVal") FALSE ("NewVal") FALSE ("NewVal") FALSE ("NewVal") FALSE ("NewVal") FALSE ("NewVal") FALSE ("NewVal") FALSE ("NewVal") FALSE ("NewVal") FALSE ("NewVal") FALSE ("NewVal") FALSE ("NewVal") FALSE ("NewVal") FALSE ("NewVal") FALSE ("NewVal") FALSE ("NewVal") FALSE ("NewVal") FALSE ("NewVal") FALSE ("NewVal") FALSE ("NewVal") FALSE ("NewVal") FALSE ("NewVal") FALSE ("NewVal") FALSE ("NewVal") FALSE ("NewVal") FALSE ("NewVal") FALSE ("NewVal") FALSE ("NewVal") FALSE ("NewVal") FALSE ("NewVal") FALSE ("NewVal") FALSE ("NewVal") FALSE ("NewVal") FALSE ("NewVal") FALSE ("NewVal") FALSE ("NewVal") FALSE ("NewVal") FALSE ("NewVal") FALSE ("NewVal") FALSE ("NewVal") FALSE ("NewVal") FALSE ("NewVal") FALSE ("NewVal") FALSE ("NewVal") FALSE ("NewVal") FALSE ("NewVal") FALSE ("NewVal") FALSE ("NewVal") FALSE ("NewVal") FALSE ("NewVal") FALSE ("NewVal") FALSE ("NewVal") FALSE ("NewVal") FALSE ("NewVal") FALSE ("NewVal") FALSE ("NewVal") FALSE ("NewVal") FALSE ("NewVal") FALSE ("NewVal") FALSE ("NewVal") FALSE ("NewVal") FALSE ("NewVal")] -> w339
          event Timeout {
            n666 = event-data() -> ()  [unwired: 1 in, 2 out]
          }
          event "RecordSel": Value Change {
            n667 = event-data() -> ("NewVal"=w342:string)  [unwired: 1 in, 4 out]
            n668 = local read "DatabaseUDL"() -> (w345:path)
            n669 = call "FeedbackDecode_UpdateDatabase.vi"("RecordsSelection"=w342, "CallType"=enum16{"Initialize", "Save", "Load"}."Load", "DatabaseUDL"=w345) -> ("DatabaseOut"=w343:T12)  [unwired: 1 in, 2 out]
            n670 = local write "Database"(w343) -> ()
          }
          event "SendComment": Value Change {
            n671 = event-data() -> ("NewVal"=w347:bool)  [unwired: 1 in, 4 out]
            n672 = case shown="True" w347 {
              frame False {
              }
              frame True {
                n673 = stacked-sequence {
                  frame #0 {
                    n674 = local read "LoopCnt"() -> (w356:u64)
                    n675 = local read "NIPTime"() -> (w352:dbl)
                    n676 = local read "Comment"() -> (w359:string)
                    n677 = Format Into String(w356) -> (resulting string=w348:string)  [unwired: 3 in, 1 out]
                    n678 = call-poly "FeedbackDecode_VariablesToString.vi"("Format"="%0.0f", "ValueIn"=w352, "FieldName"="NIPTime" ("Key Word")) -> ("StringOut"=w349:string)  [unwired: 4 in]
                    n679 = Concatenate Strings("SendComment:SS.EventID=" ("string"), w348) -> (w355:string)
                    n680 = local read "EventParamsFID"() -> (w354:refnum<file>)
                    n681 = Concatenate Strings(w355, ";SS.Comment='" ("string"), w359, "';" ("string"), w349) -> (w353:string)
                    n682 = call "FeedbackDecode_WriteTextEOL.vi"("text"=w353, "refnum in"=w354) -> ()  [unwired: 8 in, 2 out]
                  }
                  frame #1 {
                    n683 = local write "SendComment"(FALSE ("SendComment")) -> ()
                    n684 = local write "Comment"("" ("Comment")) -> ()
                  }
                }
              }
            }
          }
          event Value Change {
            n685 = event-data() -> ("NewVal"=w364:bool)  [unwired: 1 in, 4 out]
            n686 = case shown="True" w364 {
              tunnel: [FALSE ("NewVal") FALSE ("NewVal")] -> w363
              frame False {
                n687 = local read "LoopCnt"() -> (w376:u64)
                n688 = local read "NIPTime"() -> (w369:dbl)
                n689 = Format Into String(w376) -> (resulting string=w365:string)  [unwired: 3 in, 1 out]
                n690 = call-poly "FeedbackDecode_VariablesToString.vi"("Format"="%0.0f", "ValueIn"=w369, "FieldName"="NIPTime" ("Key Word")) -> ("StringOut"=w366:string)  [unwired: 4 in]
                n691 = Concatenate Strings("StopTraining:SS.EventID=" ("string"), w365) -> (w375:string)
                n692 = local read "EventParamsFID"() -> (w373:refnum<file>)
                n693 = Concatenate Strings(w375, ";SS.AcqTraining=0;" ("EventStr"), w366) -> (w372:string)
                n694 = local read "DecodeClust"() -> (w384:T5)
                n695 = call "FeedbackDecode_WriteTextEOL.vi"("text"=w372, "refnum in"=w373) -> ()  [unwired: 8 in, 2 out]
                n696 = Bundle By Name(cluster=w384, "EventStr"=w372) -> (w371:T5)
                n697 = call "FeedbackDecode_MLComCtrl.vi"("DecodeClustIn"=w371, "Mode"=T19."SendEvent") -> ("DecodeClustOut"=w370:T5)  [unwired: 6 in, 3 out]
                n698 = Unbundle By Name(w370) -> ("CtrlButtons.StartTrials"=w381:bool)
                n699 = And(x=w381, y=FALSE) -> (x .and. y?=w379:bool)
                n700 = property on="StartTrials" class="Bool (strict)"("Value"=w379) -> (error out=w378:errorcluster)  [unwired: 2 in, 1 out]
                n701 = property on="ApplyBaseline" class="Bool (strict)"(error in=w378, "DisabledEnum"=T17."Enabled" ("Disabled")) -> ()  [unwired: 1 in, 2 out]
              }
              frame True {
                n702 = local read "NIPTime"() -> (w391:dbl)
                n703 = local read "LoopCnt"() -> (w400:u64)
                n704 = call-poly "FeedbackDecode_VariablesToString.vi"("Format"="%0.0f", "ValueIn"=w391, "FieldName"="NIPTime" ("Key Word")) -> ("StringOut"=w388:string)  [unwired: 4 in]
                n705 = Format Into String(w400) -> (resulting string=w387:string)  [unwired: 3 in, 1 out]
                n706 = local read "EventParamsFID"() -> (w397:refnum<file>)
                n707 = Concatenate Strings("StartTraining:SS.EventID=" ("string"), w387) -> (w399:string)
                n708 = Concatenate Strings(w399, ";SS.AcqTraining=1;" ("EventStr"), w388) -> (w396:string)
                n709 = local read "DecodeClust"() -> (w406:T5)
                n710 = call "FeedbackDecode_WriteTextEOL.vi"("text"=w396, "refnum in"=w397) -> ()  [unwired: 8 in, 2 out]
                n711 = Bundle By Name(cluster=w406, "EventStr"=w396) -> (w395:T5)
                n712 = call "FeedbackDecode_MLComCtrl.vi"("DecodeClustIn"=w395, "Mode"=T19."SendEvent") -> ("DecodeClustOut"=w394:T5)  [unwired: 6 in, 3 out]
                n713 = Unbundle By Name(w394) -> ("ReTrain"=w407:bool)
                n714 = case shown="True" w407 {
                  tunnel: [w410 w412] -> w393
                  frame False {
                    n715 = property on="KinSrc" class="Enum (strict)"("Val(Sgnl)"=enum16{"Off", "Training", "Decode", "COB"}."Training" ("Value (Signaling)")) -> (error out=w410:errorcluster)  [unwired: 2 in, 1 out]
                  }
                  frame True {
                    n716 = property on="KinSrc" class="Enum (strict)"("Val(Sgnl)"=enum16{"Off", "Training", "Decode", "COB"}."Decode" ("Value (Signaling)")) -> (error out=w412:errorcluster)  [unwired: 2 in, 1 out]
                  }
                }
                n717 = property on="TestType" class="Enum (strict)"(error in=w393, "Val(Sgnl)"=T23."MSMS" ("Value (Signaling)")) -> (error out=w392:errorcluster)  [unwired: 1 in, 1 out]
                n718 = property on="StartTrials" class="Bool (strict)"(error in=w392, "Val(Sgnl)"=TRUE ("Value (Signaling)")) -> (error out=w402:errorcluster)  [unwired: 1 in, 1 out]
                n719 = property on="ApplyBaseline" class="Bool (strict)"(error in=w402, "DisabledEnum"=T17."Disabled and Grayed Out" ("Disabled")) -> ()  [unwired: 1 in, 2 out]
              }
            }
          }
          event Value Change {
            n720 = event-data() -> ("NewVal"=w414:bool)  [unwired: 1 in, 5 out]
            n721 = case shown="True" w414 {
              frame False {
                n722 = local read "LoopCnt"() -> (w425:u64)
                n723 = local read "NIPTime"() -> (w419:dbl)
                n724 = Format Into String(w425) -> (resulting string=w415:string)  [unwired: 3 in, 1 out]
                n725 = call-poly "FeedbackDecode_VariablesToString.vi"("Format"="%0.0f", "ValueIn"=w419, "FieldName"="NIPTime" ("Key Word")) -> ("StringOut"=w416:string)  [unwired: 4 in]
                n726 = Concatenate Strings("StopAcqBaseline:SS.EventID=" ("string"), w415) -> (w424:string)
                n727 = local read "EventParamsFID"() -> (w422:refnum<file>)
                n728 = local read "DecodeClust"() -> (w428:T5)
                n729 = Concatenate Strings(w424, ";SS.AcqBaseline=0;" ("EventStr"), w416) -> (w421:string)
                n730 = call "FeedbackDecode_WriteTextEOL.vi"("text"=w421, "refnum in"=w422) -> ()  [unwired: 8 in, 2 out]
                n731 = Bundle By Name(cluster=w428, "EventStr"=w421) -> (w420:T5)
                n732 = call "FeedbackDecode_MLComCtrl.vi"("DecodeClustIn"=w420, "Mode"=T19."SendEvent") -> ()  [unwired: 6 in, 4 out]
              }
              frame True {
                n733 = local read "LoopCnt"() -> (w439:u64)
                n734 = local read "NIPTime"() -> (w433:dbl)
                n735 = Format Into String(w439) -> (resulting string=w429:string)  [unwired: 3 in, 1 out]
                n736 = Concatenate Strings("StartAcqBaseline:SS.EventID=" ("string"), w429) -> (w438:string)
                n737 = call-poly "FeedbackDecode_VariablesToString.vi"("Format"="%0.0f", "ValueIn"=w433, "FieldName"="NIPTime" ("Key Word")) -> ("StringOut"=w430:string)  [unwired: 4 in]
                n738 = local read "EventParamsFID"() -> (w436:refnum<file>)
                n739 = local read "DecodeClust"() -> (w442:T5)
                n740 = Concatenate Strings(w438, ";SS.AcqBaseline=1;" ("EventStr"), w430) -> (w435:string)
                n741 = call "FeedbackDecode_WriteTextEOL.vi"("text"=w435, "refnum in"=w436) -> ()  [unwired: 8 in, 2 out]
                n742 = Bundle By Name(cluster=w442, "EventStr"=w435) -> (w434:T5)
                n743 = call "FeedbackDecode_MLComCtrl.vi"("DecodeClustIn"=w434, "Mode"=T19."SendEvent") -> ()  [unwired: 6 in, 4 out]
              }
            }
          }
          event "Exclude SE": Value Change {
            n744 = event-data() -> ("NewVal"=w444:bool)  [unwired: 1 in, 5 out]
            n745 = case shown="True" w444 {
              frame False {
                n746 = local read "LoopCnt"() -> (w455:u64)
                n747 = local read "NIPTime"() -> (w449:dbl)
                n748 = Format Into String(w455) -> (resulting string=w445:string)  [unwired: 3 in, 1 out]
                n749 = call-poly "FeedbackDecode_VariablesToString.vi"("Format"="%0.0f", "ValueIn"=w449, "FieldName"="NIPTime" ("Key Word")) -> ("StringOut"=w446:string)  [unwired: 4 in]
                n750 = Concatenate Strings("ExcludeSE:SS.EventID=" ("string"), w445) -> (w454:string)
                n751 = local read "EventParamsFID"() -> (w452:refnum<file>)
                n752 = local read "DecodeClust"() -> (w458:T5)
                n753 = Concatenate Strings(w454, ";SS.ExcludeSE=0;" ("EventStr"), w446) -> (w451:string)
                n754 = call "FeedbackDecode_WriteTextEOL.vi"("text"=w451, "refnum in"=w452) -> ()  [unwired: 8 in, 2 out]
                n755 = Bundle By Name(cluster=w458, "EventStr"=w451) -> (w450:T5)
                n756 = call "FeedbackDecode_MLComCtrl.vi"("DecodeClustIn"=w450, "Mode"=T19."SendEvent") -> ()  [unwired: 6 in, 4 out]
              }
              frame True {
                n757 = local read "LoopCnt"() -> (w469:u64)
                n758 = local read "NIPTime"() -> (w463:dbl)
